vi "MDF4 Close File.vi"(7 "path in":path, 8 "Error In":errorcluster, 11 "MDF4 File Reference in":i64) -> (0 "Error Out":errorcluster, 3 "MDF4 File Reference out":i64)   [LabVIEW 2019, in "MD4Logger Engine.lvlib"]
uses:
  MD4Logger Engine.lvlib
panel:
  out "error":i32
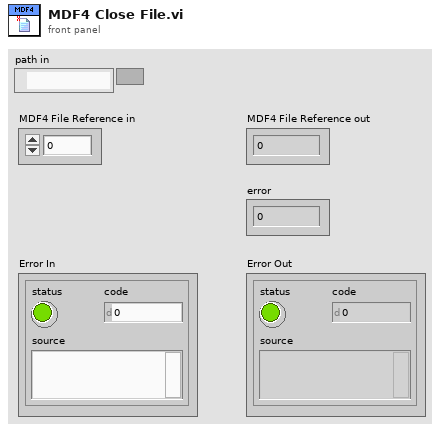
[diagram p1: front panel]
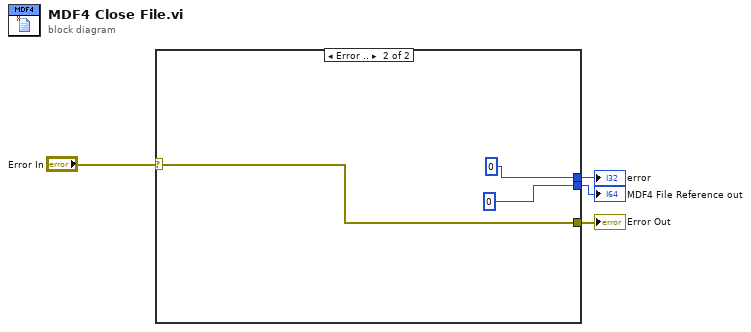
[diagram p0: block diagram]
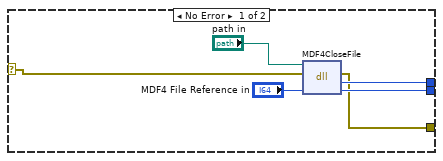
[diagram p2: hidden frame]
diagram:
  n1 = case shown="Error .." "Error In" {
    selector: "Error In" -> [w5 w13]
    tunnel: [w10 0 ("return type")] -> w4
    tunnel: [w8 i64 0 ("m4")] -> w3
    tunnel: [w6 w13] -> w2
    frame No Error {
      n2 = dll-call lib="C:/Users/Hovhannes/Desktop/MDF4API/DLL/WriterExample.dll" fn="MDF4CloseFile"(path in="path in", error in=w5, "m4"="MDF4 File Reference in") -> (error out=w6:errorcluster, "return type"=w10:i32, "m4"=w8:i64)  [unwired: 1 in, 1 out]
    }
    frame Error {
    }
  }
  "MDF4 File Reference out" <- w3
  "error" <- w4
  "Error Out" <- w2
